vi "Auo Align.vi"(1 "Noodle?":bool, 2 "RotateRight":bool, 3 "RotateLeft":bool) -> (0 "output cluster":T1)   [LabVIEW 2014]
uses:
  TypeDefs/SRE Enum.ctl
panel:
  in  "Gyro Tolerance":dbl=2.0 format="%#_13g"
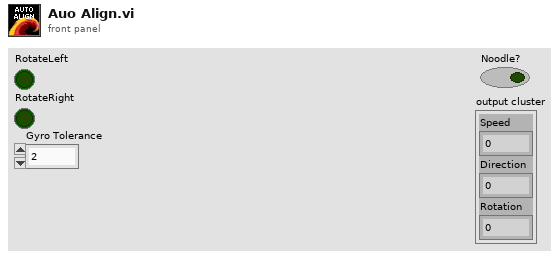
[diagram p1: front panel]
types:
  T1 = cluster{"Speed":dbl, "Direction":dbl, "Rotation":dbl}
  T2 = typedef "SRE Enum.ctl" = enum16{"Start", "Run", "End"}
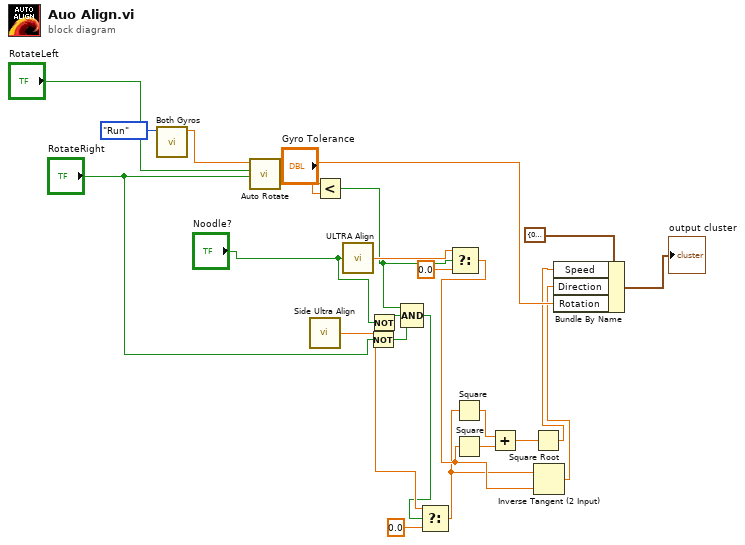
[diagram p0: block diagram]
diagram:
  n1 = call "Both Gyros.vi"("Enum"=SRE_Enum."Run") -> ("Angle"=w24:dbl)  [unwired: 10 in]
  n2 = call "Auto Rotate.vi"("RotateRight"="RotateRight", "RotateLeft"="RotateLeft", "Gyroscope"=w24) -> ("Rotation Speed"=w19:dbl)  [unwired: 8 in]
  n3 = call "Side Ultra Align.vi"() -> ("Speed"=w9:dbl)  [unwired: 1 in]
  n4 = Less?(x=w19, y="Gyro Tolerance") -> (x < y?=w7:bool)
  n5 = call "ULTRA Align.vi"("Noodle?"="Noodle?") -> ("Speed"=w14:dbl)
  n6 = Not(x="RotateRight") -> (.not. x?=w3:bool)
  n7 = Not(x="Noodle?") -> (.not. x?=w6:bool)
  n8 = Compound Arithmetic op=AND(w7, w6, w3) -> (w4:bool)
  n9 = Select(t=w9, s=w4, f=0.0) -> (s? t:f=w8:dbl)
  n10 = Select(t=w14, s=w7, f=0.0) -> (s? t:f=w13:dbl)
  n11 = Square(x=w8) -> (x^2=w16:dbl)
  n12 = Square(x=w13) -> (x^2=w17:dbl)
  n13 = Add(x=w16, y=w17) -> (x+y=w15:dbl)
  n14 = Square Root(x=w15) -> (sqrt(x)=w11:dbl)
  n15 = Inverse Tangent (2 Input)(1:w13, 2:w8) -> (0:w12:dbl)
  n16 = Bundle By Name(cluster=T1 {"Speed"=0.0, "Direction"=0.0, "Rotation"=0.0} ("output cluster"), "Speed"=w11, "Direction"=w12, "Rotation"=w19) -> (→"output cluster":T1)
